vi "Get UIAs prefixes.vi"(11 "DualScreenH in":refnum<class "DualScreenH.lvclass">) -> (2 "2nd UIA prefix":string, 3 "1st UIA prefix":string)   [LabVIEW 2020, in "DualScreenH.lvlib" / "DualScreenH.lvclass"]
uses:
  DualScreenH.lvclass
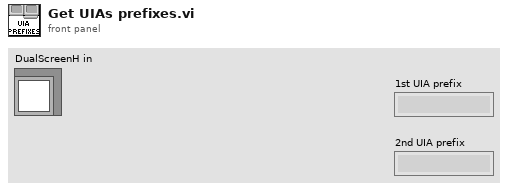
[diagram p1: front panel]
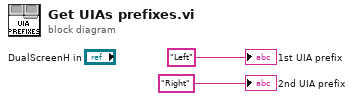
[diagram p0: block diagram]
diagram:
  "1st UIA prefix" <- "Left" ("String")
  "2nd UIA prefix" <- "Right" ("String")
